vi "check source version.vi"() -> (2 "application name":string, 3 "year":i32, 4 "Newer version available":bool, 5 "continue running?":bool)   [LabVIEW 2015]
uses:
  version state.ctl
panel:
  out "version state":T1
  out "this version":path
  out "This version":timestamp
  out "time stamp":timestamp
  out "Connection":string
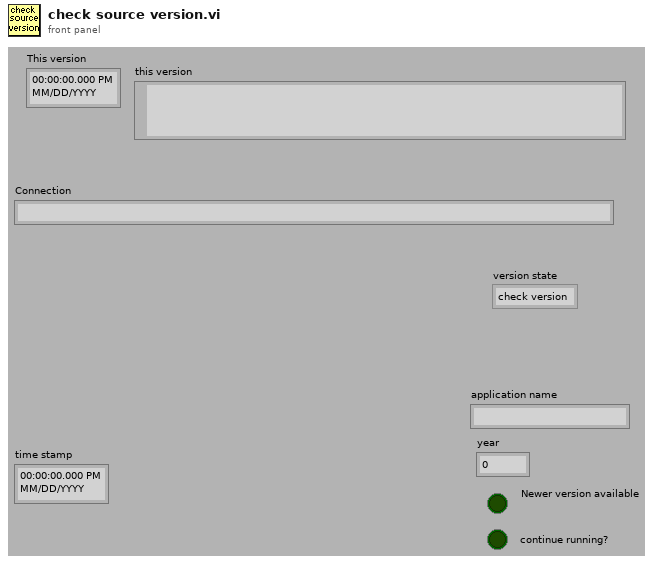
[diagram p1: front panel]
types:
  T1 = typedef "version state.ctl" = enum16{"check version", "prompt for update", "go to download", "accept license", "display copyright", "done"}
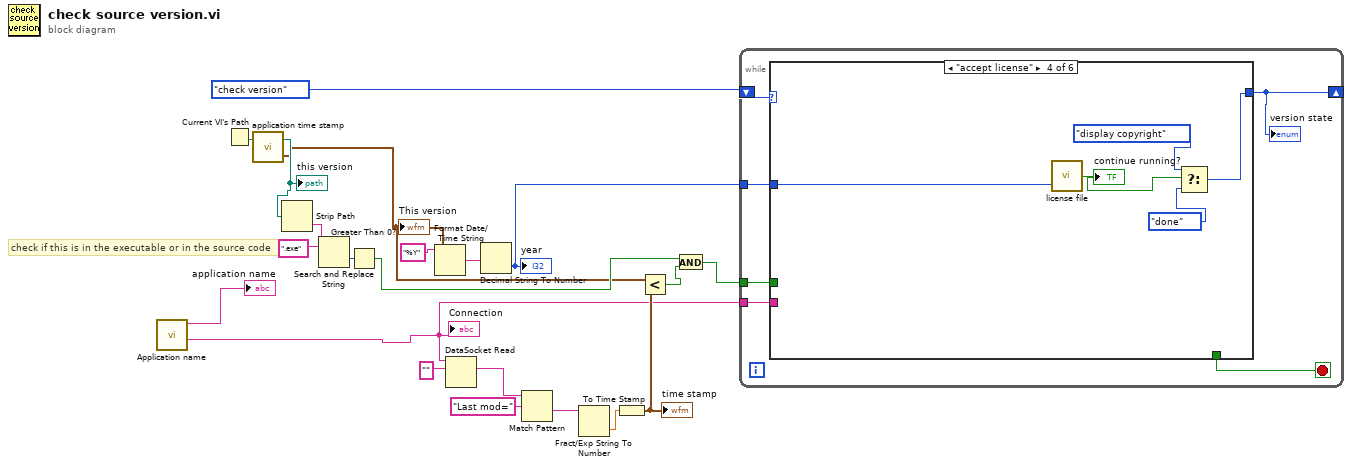
[diagram p0: block diagram]
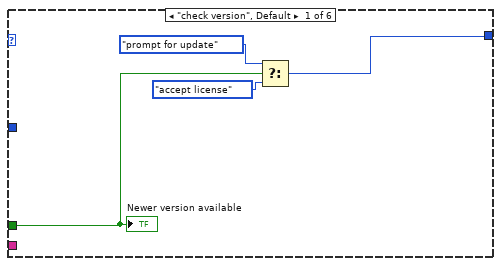
[diagram p2: hidden frame]
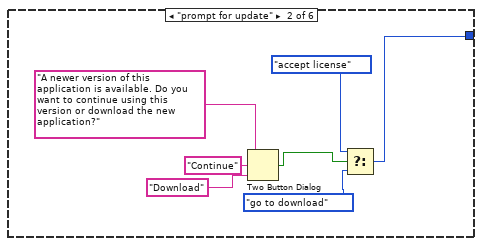
[diagram p3: hidden frame]
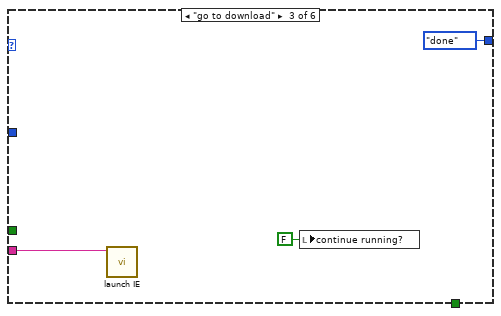
[diagram p4: hidden frame]
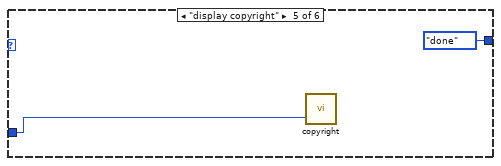
[diagram p5: hidden frame]
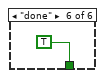
[diagram p6: hidden frame]
diagram:
  # "check if this is in the executable or in the source code"
  n1 = call "Application name.vi"() -> ("download site"=w4:string, "application name"=→"application name":string)  [unwired: 5 in, 1 out]
  "Connection" <- w4
  n2 = Current VI's Path() -> (path=w3:path)
  n3 = call "application time stamp.vi"("VI Path"=w3) -> ("last mod"=w1:timestamp, "this version"=w2:path)  [unwired: 1 in]
  "This version" <- w1
  "this version" <- w2
  n4 = Strip Path(path=w2) -> (name=w10:string)  [unwired: 1 out]
  n5 = Search and Replace String(input string=w10, search string=".exe") -> (offset past replacement=w11:i32)  [unwired: 6 in, 3 out]
  n6 = Greater Than 0?(x=w11) -> (x > 0?=w9:bool)
  n7 = Format Date/Time String(time format string (%c)="%Y", seconds (now)=w1) -> (date/time string=w21:string)  [unwired: 1 in]
  n8 = DataSocket Read(10:"" ("text"), 11:w4) -> (2:w15:string)  [unwired: 3 in, 6 out]
  n9 = Decimal String To Number(string=w21) -> (number=w14:i32)  [unwired: 2 in, 1 out]
  "year" <- w14
  n10 = Match Pattern(string=w15, regular expression="Last mod=") -> (after substring=w17:string)  [unwired: 1 in, 3 out]
  n11 = Fract/Exp String To Number(string=w17) -> (number=w18:dbl)  [unwired: 3 in, 1 out]
  n12 = To Time Stamp(1:w18) -> (0:w19:timestamp)
  "time stamp" <- w19
  n13 = Less?(x=w1, y=w19) -> (x < y?=w8:bool)
  n14 = And(x=w9, y=w8) -> (x .and. y?=w7:bool)
  n15 = while {
    shift-right: [w27] -> _
    shift-left: version_state."check version" ("version state") -> [w26]
    tunnel: w7 -> [w25]
    tunnel: w4 -> [w24]
    tunnel: w14 -> [w23]
    stop <- w22 stop-if-true
    n16 = case shown="\"accept license\"" w26 {
      tunnel: [w31 w32 version_state."done" ("version state") w43 version_state."done" ("version state") _] -> w27
      tunnel: w25 -> [w28 _ _ _ _ _]
      tunnel: w24 -> [_ _ w40 _ _ _]
      tunnel: w23 -> [_ _ _ w46 w48 _]
      tunnel: [_ _ _ _ _ TRUE] -> w22
      frame "check version", Default {
        n17 = Select(t=version_state."prompt for update" ("version state"), s=w28, f=version_state."accept license" ("version state")) -> (s? t:f=w31:T1)
        "Newer version available" <- w28
      }
      frame "prompt for update" {
        n18 = Two Button Dialog(message="A newer version of this application is available. Do you want to continue using this version or download the new application?", 1:"Download" ("F button name (\"Cancel\")"), 2:"Continue" ("T button name (\"OK\")")) -> (T button?=w35:bool)
        n19 = Select(t=version_state."accept license" ("version state"), s=w35, f=version_state."go to download" ("version state")) -> (s? t:f=w32:T1)
      }
      frame "go to download" {
        n20 = call "launch IE.vi"("web site"=w40) -> ()  [unwired: 10 in, 1 out]
        n21 = local write "continue running?"(FALSE ("continue running?")) -> ()
      }
      frame "accept license" {
        n22 = call "license file.vi"("year"=w46) -> ("Accepted"=w45:bool)  [unwired: 1 in]
        "continue running?" <- w45
        n23 = Select(t=version_state."display copyright" ("version state"), s=w45, f=version_state."done" ("version state")) -> (s? t:f=w43:T1)
      }
      frame "display copyright" {
        n24 = call "copyright.vi"("year"=w48) -> ()  [unwired: 3 in]
      }
      frame "done" {
      }
    }
    "version state" <- w27
  }
